vi "number1_sub1-configure data acquisition.vi"(5 "OK Button":bool) -> ()   [LabVIEW 2014]
uses:
  number1_global.vi
panel:
  in  "samples per acquisition":dbl=10000.0
  in  "sampling rate (samples/sec)":dbl=1000.0
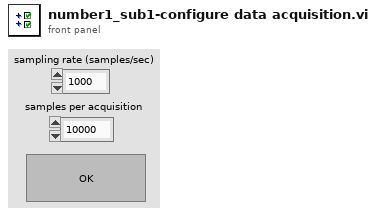
[diagram p1: front panel]
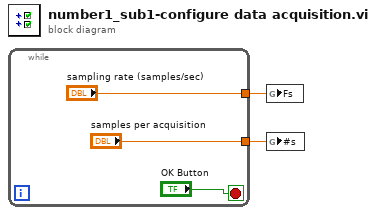
[diagram p0: block diagram]
diagram:
  n1 = while {
    tunnel: ["sampling rate (samples/sec)"] -> w2
    tunnel: ["samples per acquisition"] -> w1
    stop <- "OK Button" stop-if-true
  }
  n2 = global write "number1_global.vi" "Fs"(w2) -> ()
  n3 = global write "number1_global.vi" "#s"(w1) -> ()
